vi "Test 1000 Log Writes.vi"(11 "Test Case In":refnum<class "Stress.lvclass">) -> (0 "error out":errorcluster, 3 "Test Case Out":refnum<class "Stress.lvclass">)   [LabVIEW 2020]
uses:
  Stress/Stress.lvclass
  C:/Program Files (x86)/National Instruments/LabVIEW 2020/vi.lib/Astemes/LUnit/Test Case.lvclass
  Source/Type Defs/Debug Level.ctl
  <vilib>/Astemes/LUnit/Test Case.lvclass/Test Case.ctl
  4993e8ee-a06a-463a-9684-69129f64d5ce.vi
  <vilib>/Astemes/LUnit/Core/LUnit Test Case/Private/Append Pass Result.vi
  <vilib>/Astemes/LUnit/Core/LUnit Test Case/Private/Append Fail Result.vi
  4993e8ee-a06a-463a-9684-69129f64d5ce.vi/9c5d11cd-9439-4240-a1ee-d9baace9c924.vi
  <vilib>/Astemes/LUnit/Core/LUnit Test Case/Private/Run In UI.vi
  <vilib>/Utility/error.llb/Clear Errors.vi
  Source/Sinks/File Sink/File Sink.lvclass
  C:/Users/hughe_cx/Documents/05_repos/LVLog/Source/Sinks/Sink/Sink.lvclass
  Source/LV Log.lvlib
  Source/Logger/Logger.lvclass
  Testing.lvlib
  <vilib>/Astemes/LUnit/Test Case.lvclass
panel:
  out "Iteration (of 10000)":i32
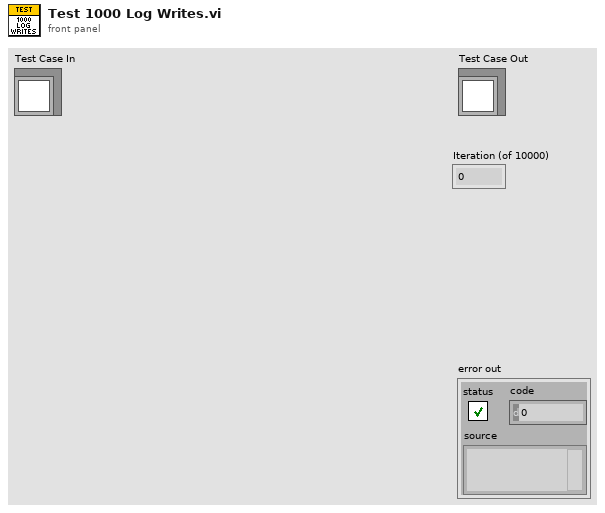
[diagram p1: front panel]
types:
  T1 = typedef "LV Log.lvlib/Debug Level.ctl" = enum16{"DEFAULT", "DEBUG", "INFO", "WARN", "ERROR", "FATAL"}
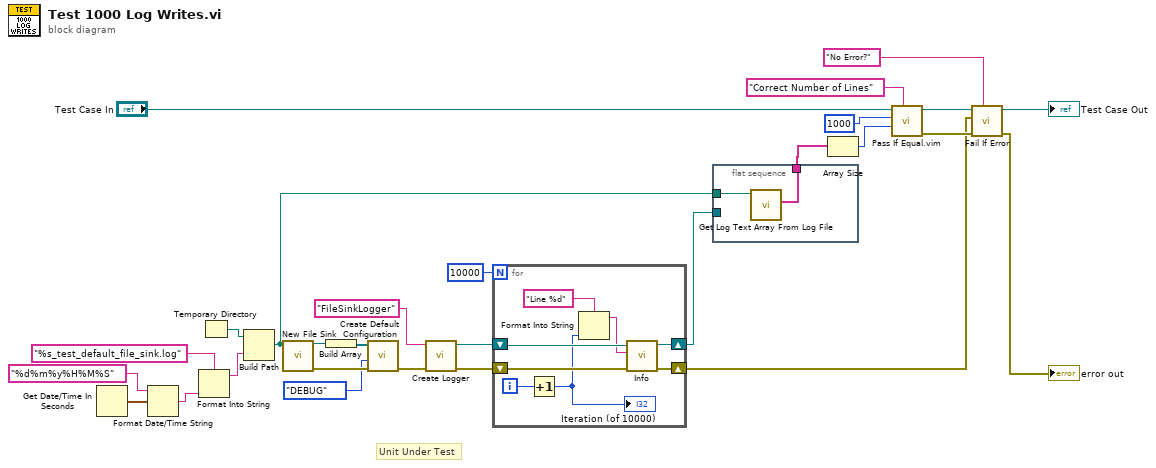
[diagram p0: block diagram]
diagram:
  # "Unit Under Test"
  n1 = Get Date/Time In Seconds() -> (seconds since 1Jan1904=w20:timestamp)
  n2 = Format Date/Time String(time format string (%c)="%d%m%y%H%M%S", seconds (now)=w20) -> (date/time string=w18:string)  [unwired: 1 in]
  n3 = Format Into String(format string="%s_test_default_file_sink.log", w18) -> (resulting string=w21:string)  [unwired: 2 in, 1 out]
  n4 = Temporary Directory() -> (w23:path)
  n5 = Build Path(base path=w23, name or relative path=w21) -> (appended path=w12:path)
  n6 = call "New File Sink.vi"("File Path"=w12) -> ("error out"=w26:errorcluster, "File Sink out"=w24:refnum<class "File Sink.lvclass">)  [unwired: 9 in]
  n7 = Build Array(w24) -> (w25:refnum<class "File Sink.lvclass">[])
  n8 = call "Create Default Configuration.vi"("Sinks"=w25, "Debug Level in"=Debug_Level."DEBUG", "error in (no error)"=w26) -> ("error out"=w27:errorcluster)  [unwired: 7 in]
  n9 = call "Create Logger.vi"("error in (no error)"=w27, "Name"="FileSinkLogger") -> ("error out"=w16:errorcluster, "Logger out"=w15:refnum<class "Logger.lvclass">)  [unwired: 8 in]
  n10 = for {
    N: 10000 -> [_]
    shift-right: [w33] -> w11
    shift-left: w15 -> [w35]
    shift-right: [w34] -> w3
    shift-left: w16 -> [w36]
    i -> [w30]
    n11 = Increment(x=w30) -> (x+1=w29:i32)
    "Iteration (of 10000)" <- w29
    n12 = Format Into String(format string="Line %d" ("Log Text"), w29) -> (resulting string=w31:string)  [unwired: 2 in, 1 out]
    n13 = call "Info.vi"("error in (no error)"=w36, "Log Text"=w31, "Logger in"=w35) -> ("error out"=w34:errorcluster, "Logger out"=w33:refnum<class "Logger.lvclass">)  [unwired: 6 in, 1 out]
  }
  n14 = flat-sequence {
    tunnel: [w38] -> w10
    tunnel: w12 -> [w37]
    tunnel: w11 -> [_]
    frame #0 {
      n15 = call "Get Log Text Array From Log File.vi"("Log File Path in"=w37) -> ("Log Text Array"=w38:string[])  [unwired: 8 in, 2 out]
    }
  }
  n16 = Array Size(array=w10) -> (size(s)=w9:i32)
  n17 = call "Pass If Equal.vim"("Description"="Correct Number of Lines", "Actual"=w9, "Expected"=1000, "LUnit Test Case In"="Test Case In") -> ("error out"=w6:errorcluster, "LUnit Test Case Out"=w5:refnum<class "Stress.lvclass">)  [unwired: 6 in]
  n18 = call <vilib>:"Fail If Error.vi"("Description"="No Error?", "error in (no error)"=w6, "Assert error"=w3, "LUnit Test Case In"=w5) -> ("error out"=→"error out":errorcluster, "LUnit Test Case Out"=→"Test Case Out":refnum<class "Stress.lvclass">)  [unwired: 6 in]
